vi "Find all UI Control Type Classes.vi"(4 "Label Black List":string[](array[string]), 5 "Reset to Defaults":bool, 6 "Label White List":string[](array[string]), 7 "Tab Label in Tag?":bool, 8 "error in (no error)":errorcluster, 9 "Root Label":string, 10 "Ctl Refnum":refnum<vi>, 11 "VI in":refnum<vi>) -> (0 "error out":errorcluster, 1 "Labels":string[](array[string]), 3 "Values":refnum<class "Abs_Type.lvclass">[](array[class]))   [LabVIEW 2021, in "UI-Bus.lvclass"]
uses:
  UI-Bus.lvclass
  <vilib>/TSA/Abstract Data Classes/Abs_Types/Type/Abs_Type.lvclass
  Support/Boolean/UI-Bus_Boolean.lvclass
  C:/Program Files (x86)/National Instruments/LabVIEW 2021/vi.lib/TSA/Abstract Data Classes/Abs_Types/Type/Abs_Type.lvclass
  C:/Program Files (x86)/National Instruments/LabVIEW 2021/vi.lib/TSA/Abstract Data Classes/Abs_Types/Value/Abs_Value.lvclass
  Support/U8/UI-Bus_U8.lvclass
  C:/Program Files (x86)/National Instruments/LabVIEW 2021/vi.lib/TSA/Abstract Data Classes/Abs_Types/Numeric/Abs_Numeric.lvclass
  Support/U16/UI-Bus_U16.lvclass
  Support/U32/UI-Bus_U32.lvclass
  Support/U64/UI-Bus_U64.lvclass
  Support/I8/UI-Bus_I8.lvclass
  Support/I16/UI-Bus_I16.lvclass
  Support/I32/UI-Bus_I32.lvclass
  Support/I64/UI-Bus_I64.lvclass
  Support/Single/UI-Bus_Single.lvclass
  Support/Double/UI-Bus_Double.lvclass
  Support/Extended/UI-Bus_Extended.lvclass
  Support/Complex Single/UI-Bus_ComplexSingle.lvclass
  Support/Complex Double/UI-Bus_ComplexDouble.lvclass
  Support/Complex Extended/UI-Bus_ComplexExtended.lvclass
  Support/Time/UI-Bus_Time.lvclass
  Support/String/UI-Bus_String.lvclass
  Support/Variant/UI-Bus_Variant.lvclass
  <vilib>/TSA/Abstract Data Classes/Abs_Types/Numeric/Abs_Numeric.lvclass
  <vilib>/Utility/Data Type/NI_Data Type.lvlib
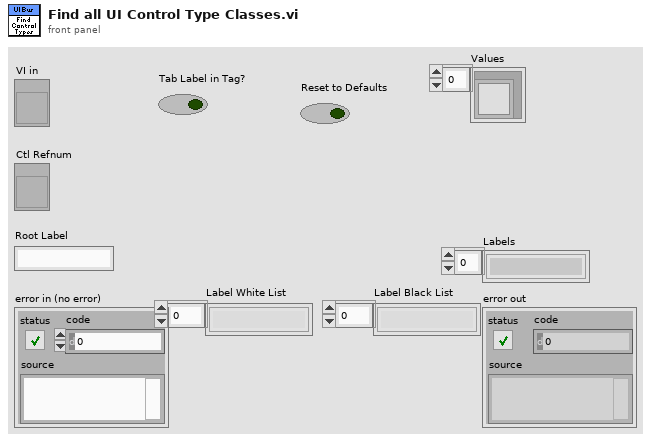
[diagram p1: front panel]
types:
  T1 = typedef "NI_Data Type.lvlib/Data Type.ctl" = enum8{"Invalid Type", "Void", "I8", "I16", "I32", "I64", "U8", "U16", "U32", "U64", "Single Float", "Double Float", "Extended Float", "Single Complex", "Double Complex", "Extended Complex", "Enum U8", "Enum U16", "Enum U32", "Enum U64", "Single Float With Unit", "Double Float With Unit", "Extended Float With Unit", "Single Complex with Unit", "Double Complex with Unit", "Extended Complex with Unit", "Boolean", "String", "Path", "Picture", "Tag", "Array", "Cluster", "Variant", "LV Variant", "Waveform", "Timestamp", "Digital Waveform", "Digital Data", "ExpressData", "Refnum", "External Data", "VI", "Poly VI", "LabVIEW Class Instance", "Fixed Point", "Set Collection", "Map Collection"}
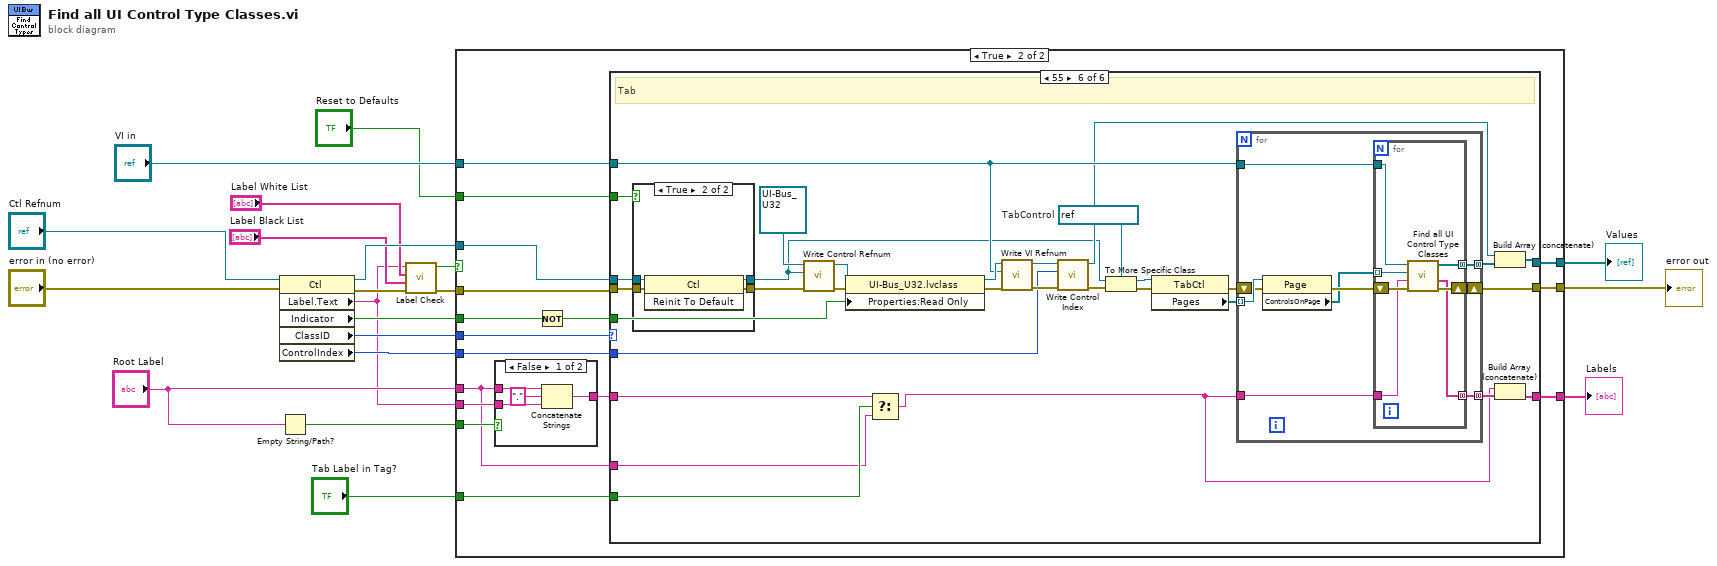
[diagram p0: block diagram]
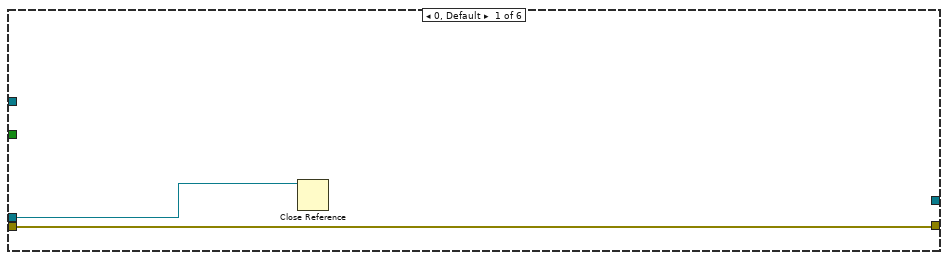
[diagram p4: hidden frame]
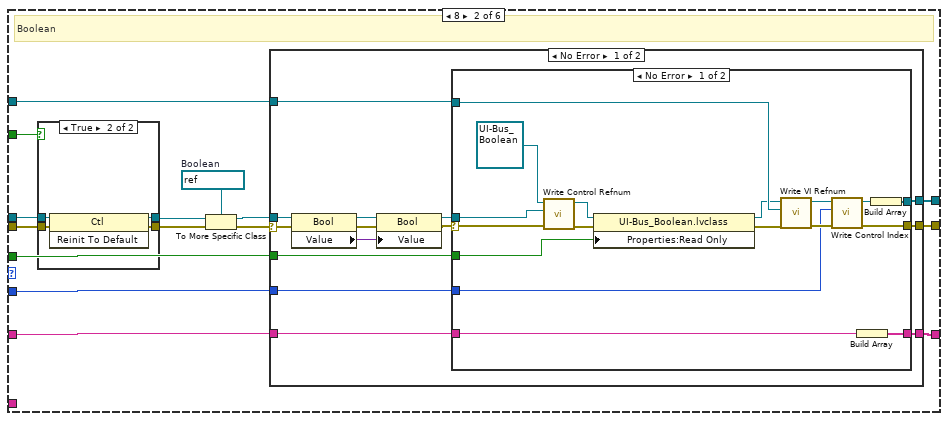
[diagram p5: hidden frame]
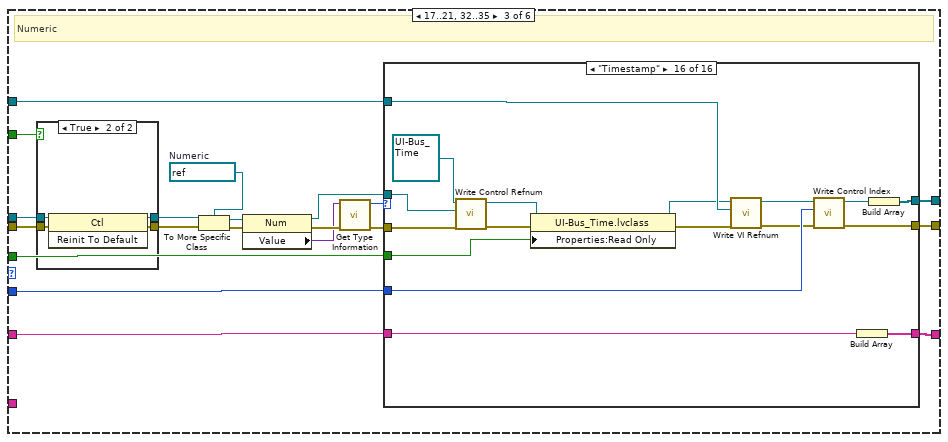
[diagram p9: hidden frame]
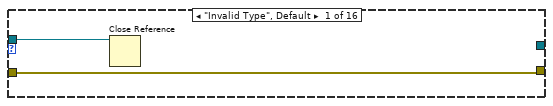
[diagram p11: hidden frame]
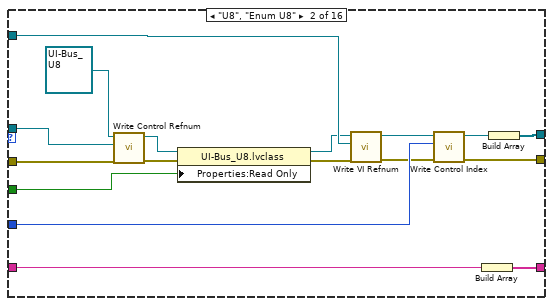
[diagram p12: hidden frame]
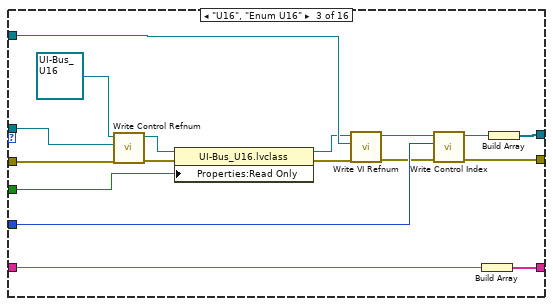
[diagram p13: hidden frame]
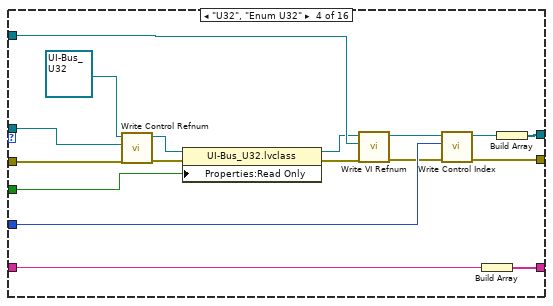
[diagram p14: hidden frame]
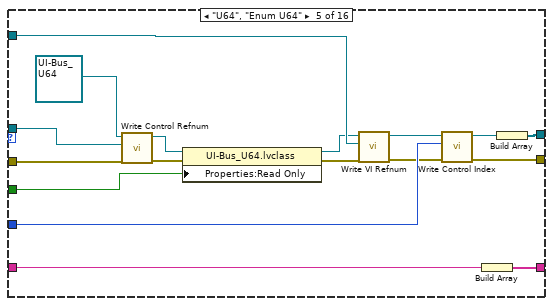
[diagram p15: hidden frame]
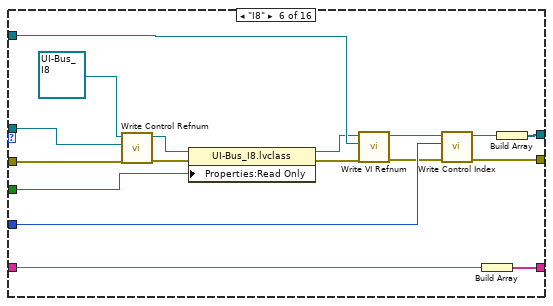
[diagram p16: hidden frame]
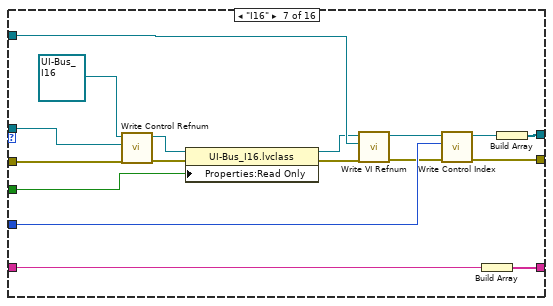
[diagram p17: hidden frame]
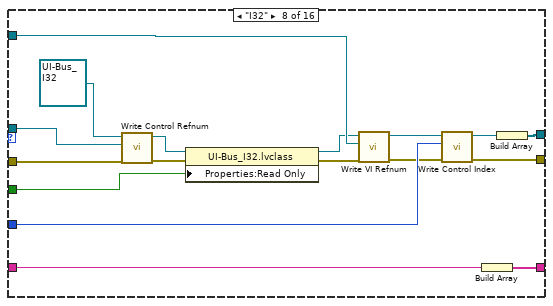
[diagram p18: hidden frame]
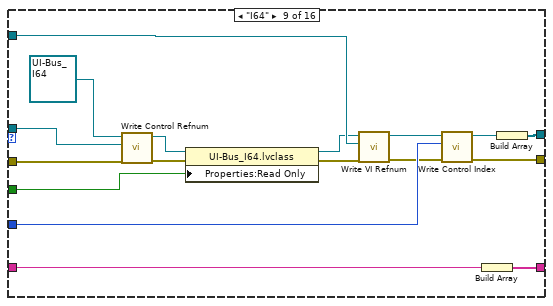
[diagram p19: hidden frame]
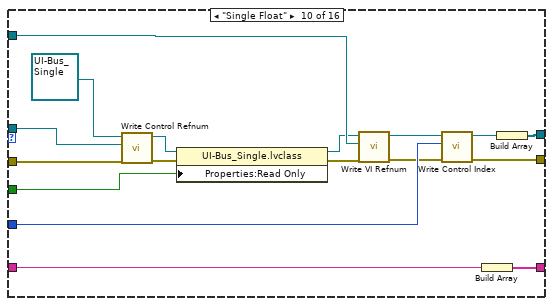
[diagram p20: hidden frame]
diagram:
  n1 = property class="Ctl"(reference="Ctl Refnum", error in="error in (no error)") -> (reference out=w19:refnum<vi>, error out=w11:errorcluster, "Label.Text"=w4:string, "Indicator"=w12:bool, "ClassID"=w13:u32, "ControlIndex"=w18:i32)
  n2 = Empty String/Path?(string/path="Root Label") -> (empty?=w15:bool)
  n3 = call "Label Check.vi"("error in (no error)"=w11, "Label Black List"="Label Black List", "Label White List"="Label White List", "Label"=w4) -> ("error out"=w10:errorcluster, "OK"=w9:bool)  [unwired: 6 in]
  n4 = case shown="True" w9 {
    tunnel: [w21 w37] -> w20
    tunnel: [_ w36] -> w5
    tunnel: w19 -> [_ w35]
    tunnel: w18 -> [_ w34]
    tunnel: "VI in" -> [_ w33]
    tunnel: [_ w32] -> w16
    tunnel: w15 -> [_ w31]
    tunnel: "Root Label" -> [_ w23]
    tunnel: w13 -> [_ w29]
    tunnel: w12 -> [_ w28]
    tunnel: w10 -> [w21 w26]
    tunnel: w4 -> [_ w24]
    tunnel: "Tab Label in Tag?" -> [_ w25]
    tunnel: "Reset to Defaults" -> [_ w22]
    frame False {
    }
    frame True {
      n5 = case shown="False" w31 {
        tunnel: w24 -> [w39 w42]
        tunnel: [w40 w42] -> w30
        tunnel: w23 -> [w38 _]
        frame False {
          n6 = Concatenate Strings(w38, "." ("string"), w39) -> (w40:string)
        }
        frame True {
        }
      }
      n7 = Not(x=w28) -> (.not. x?=w27:bool)
      n8 = case shown="55" w29 {
        tunnel: w26 -> [w44 w49 w102 w385 w411 w439]
        tunnel: w33 -> [_ w59 w117 w400 w426 w443]
        tunnel: w34 -> [_ w58 w116 w399 w425 w442]
        tunnel: w35 -> [w43 w48 w101 w384 w410 w438]
        tunnel: [_ w57 w115 w398 w424 w441] -> w36
        tunnel: [w44 w54 w112 w395 w421 w457] -> w37
        tunnel: w30 -> [_ w56 w114 w397 w423 w455]
        tunnel: [_ w55 w113 w396 w422 w434] -> w32
        tunnel: w27 -> [_ w53 w111 w394 w420 w444]
        tunnel: w25 -> [_ _ _ _ _ w454]
        tunnel: w23 -> [_ _ _ _ _ w453]
        tunnel: w22 -> [_ w45 w98 w381 w407 w435]
        frame 0, Default {
          n9 = Close Reference(reference=w43) -> ()  [unwired: 1 in, 1 out]
        }
        frame 8 {
          w52 = refnum<vi> refnum  # Boolean
          # "Boolean"
          n10 = case shown="True" w45 {
            tunnel: w49 -> [w60 w65]
            tunnel: w48 -> [w61 w64]
            tunnel: [w60 w63] -> w47
            tunnel: [w61 w62] -> w46
            frame False {
            }
            frame True {
              n11 = invoke class="Ctl" method="Reinit To Default"(reference=w64, error in=w65) -> (reference out=w62:refnum<vi>, error out=w63:errorcluster)  [unwired: 1 in, 1 out]
            }
          }
          n12 = To More Specific Class(target class=w52, reference=w46, error in=w47) -> (specific class reference=w50:refnum<vi>, error out=w51:errorcluster)
          n13 = case shown="No Error" w51 {
            selector: w51 -> [w70 w97]
            tunnel: w59 -> [w79 _]
            tunnel: w58 -> [w78 _]
            tunnel: [w77 _] -> w57
            tunnel: w56 -> [w76 _]
            tunnel: [w75 _] -> w55
            tunnel: [w74 w97] -> w54
            tunnel: w53 -> [w73 _]
            tunnel: w50 -> [w69 _]
            frame No Error {
              n14 = property class="Bool"(reference=w69, error in=w70) -> (reference out=w67:refnum<vi>, error out=w68:errorcluster, "Value"=w66:variant)
              n15 = property class="Bool"(reference=w67, error in=w68, "Value"=w66) -> (reference out=w72:refnum<vi>, error out=w71:errorcluster)
              n16 = case shown="No Error" w71 {
                selector: w71 -> [w80 _]
                tunnel: w79 -> [w96 _]
                tunnel: w78 -> [w93 _]
                tunnel: [w92 _] -> w77
                tunnel: w76 -> [w91 _]
                tunnel: [w90 _] -> w75
                tunnel: [w89 _] -> w74
                tunnel: w73 -> [w82 _]
                tunnel: w72 -> [w81 _]
                frame No Error {
                  n17 = call-dynamic "Write Control Refnum.vi"("error in (no error)"=w80, "Ctl Refnum"=w81, "UI-Bus_Boolean in"=refnum<class "UI-Bus_Boolean.lvclass"> refnum ("UI-Bus_Boolean.lvclass")) -> ("error out"=w86:errorcluster, "UI-Bus_Boolean out"=w84:refnum<class "UI-Bus_Boolean.lvclass">)  [unwired: 7 in]
                  n18 = property class="UI-Bus_Boolean.lvclass"(reference=w84, error in=w86, "Properties:Read Only"=w82) -> (reference out=w83:refnum<class "UI-Bus_Boolean.lvclass">, error out=w85:errorcluster)
                  n19 = call-dynamic "Write VI Refnum.vi"("error in (no error)"=w85, "VI Refnum"=w96, "UI-Bus_Boolean in"=w83) -> ("error out"=w95:errorcluster, "UI-Bus_Boolean out"=w94:refnum<class "UI-Bus_Boolean.lvclass">)  [unwired: 7 in]
                  n20 = call-dynamic "Write Control Index.vi"("error in (no error)"=w95, "Control Index"=w93, "UI-Bus_Boolean in"=w94) -> ("error out"=w89:errorcluster, "UI-Bus_Boolean out"=w88:refnum<class "UI-Bus_Boolean.lvclass">)  [unwired: 7 in]
                  n21 = Build Array(w91) -> (w90:string[])
                  n22 = Build Array(w88) -> (w92:refnum<class "UI-Bus_Boolean.lvclass">[])
                }
                frame Error {
                  # "If the boolean has a latching action then a reading from it will error"
                }
              }
            }
            frame Error {
            }
          }
        }
        frame 17..21, 32..35 {
          w110 = refnum<vi> refnum  # Numeric
          # "Numeric"
          n23 = case shown="True" w98 {
            tunnel: w102 -> [w118 w123]
            tunnel: w101 -> [w119 w122]
            tunnel: [w118 w121] -> w100
            tunnel: [w119 w120] -> w99
            frame False {
            }
            frame True {
              n24 = invoke class="Ctl" method="Reinit To Default"(reference=w122, error in=w123) -> (reference out=w120:refnum<vi>, error out=w121:errorcluster)  [unwired: 1 in, 1 out]
            }
          }
          n25 = To More Specific Class(target class=w110, reference=w99, error in=w100) -> (specific class reference=w108:refnum<vi>, error out=w109:errorcluster)
          n26 = property class="Num"(reference=w108, error in=w109) -> (reference out=w105:refnum<vi>, error out=w107:errorcluster, "Value"=w106:variant)
          n27 = call <vilib>:"Get Type Information.vi"("error in (no error)"=w107, "variant"=w106) -> ("error out"=w103:errorcluster, "type"=w104:T1)  [unwired: 5 in, 3 out]
          n28 = case shown="\"Timestamp\"" w104 {
            tunnel: w117 -> [_ w142 w159 w176 w193 w210 w227 w244 w261 w278 w295 w312 w329 w346 w363 w380]
            tunnel: w116 -> [_ w141 w158 w175 w192 w209 w226 w243 w260 w277 w294 w311 w328 w345 w362 w379]
            tunnel: [_ w140 w157 w174 w191 w208 w225 w242 w259 w276 w293 w310 w327 w344 w361 w378] -> w115
            tunnel: w114 -> [_ w139 w156 w173 w190 w207 w224 w241 w258 w275 w292 w309 w326 w343 w360 w377]
            tunnel: [_ w138 w155 w172 w189 w206 w223 w240 w257 w274 w291 w308 w325 w342 w359 w376] -> w113
            tunnel: [w125 w137 w154 w171 w188 w205 w222 w239 w256 w273 w290 w307 w324 w341 w358 w375] -> w112
            tunnel: w111 -> [_ w136 w153 w170 w187 w204 w221 w238 w255 w272 w289 w306 w323 w340 w357 w374]
            tunnel: w105 -> [w124 w127 w145 w162 w179 w196 w213 w230 w247 w264 w281 w298 w315 w332 w349 w366]
            tunnel: w103 -> [w125 w126 w144 w161 w178 w195 w212 w229 w246 w263 w280 w297 w314 w331 w348 w365]
            frame "Invalid Type", Default {
              n29 = Close Reference(reference=w124) -> ()  [unwired: 1 in, 1 out]
            }
            frame "U8", "Enum U8" {
              n30 = call-dynamic "Write Control Refnum.vi"("error in (no error)"=w126, "Ctl Refnum"=w127, "UI-Bus_Boolean in"=refnum<class "UI-Bus_U8.lvclass"> refnum ("UI-Bus_U8.lvclass")) -> ("error out"=w132:errorcluster, "UI-Bus_Boolean out"=w130:refnum<class "UI-Bus_U8.lvclass">)  [unwired: 7 in]
              n31 = property class="UI-Bus_U8.lvclass"(reference=w130, error in=w132, "Properties:Read Only"=w136) -> (reference out=w129:refnum<class "UI-Bus_U8.lvclass">, error out=w131:errorcluster)
              n32 = call-dynamic "Write VI Refnum.vi"("error in (no error)"=w131, "VI Refnum"=w142, "UI-Bus_Boolean in"=w129) -> ("error out"=w135:errorcluster, "UI-Bus_Boolean out"=w134:refnum<class "UI-Bus_U8.lvclass">)  [unwired: 7 in]
              n33 = call-dynamic "Write Control Index.vi"("error in (no error)"=w135, "Control Index"=w141, "UI-Bus_Boolean in"=w134) -> ("error out"=w137:errorcluster, "UI-Bus_Boolean out"=w133:refnum<class "UI-Bus_U8.lvclass">)  [unwired: 7 in]
              n34 = Build Array(w139) -> (w138:string[])
              n35 = Build Array(w133) -> (w140:refnum<class "UI-Bus_U8.lvclass">[])
            }
            frame "U16", "Enum U16" {
              n36 = call-dynamic "Write Control Refnum.vi"("error in (no error)"=w144, "Ctl Refnum"=w145, "UI-Bus_Boolean in"=refnum<class "UI-Bus_U16.lvclass"> refnum ("UI-Bus_U16.lvclass")) -> ("error out"=w149:errorcluster, "UI-Bus_Boolean out"=w147:refnum<class "UI-Bus_U16.lvclass">)  [unwired: 7 in]
              n37 = property class="UI-Bus_U16.lvclass"(reference=w147, error in=w149, "Properties:Read Only"=w153) -> (reference out=w146:refnum<class "UI-Bus_U16.lvclass">, error out=w148:errorcluster)
              n38 = call-dynamic "Write VI Refnum.vi"("error in (no error)"=w148, "VI Refnum"=w159, "UI-Bus_Boolean in"=w146) -> ("error out"=w152:errorcluster, "UI-Bus_Boolean out"=w151:refnum<class "UI-Bus_U16.lvclass">)  [unwired: 7 in]
              n39 = call-dynamic "Write Control Index.vi"("error in (no error)"=w152, "Control Index"=w158, "UI-Bus_Boolean in"=w151) -> ("error out"=w154:errorcluster, "UI-Bus_Boolean out"=w150:refnum<class "UI-Bus_U16.lvclass">)  [unwired: 7 in]
              n40 = Build Array(w156) -> (w155:string[])
              n41 = Build Array(w150) -> (w157:refnum<class "UI-Bus_U16.lvclass">[])
            }
            frame "U32", "Enum U32" {
              n42 = call-dynamic "Write Control Refnum.vi"("error in (no error)"=w161, "Ctl Refnum"=w162, "UI-Bus_Boolean in"=refnum<class "UI-Bus_U32.lvclass"> refnum ("UI-Bus_U32.lvclass")) -> ("error out"=w166:errorcluster, "UI-Bus_Boolean out"=w164:refnum<class "UI-Bus_U32.lvclass">)  [unwired: 7 in]
              n43 = property class="UI-Bus_U32.lvclass"(reference=w164, error in=w166, "Properties:Read Only"=w170) -> (reference out=w163:refnum<class "UI-Bus_U32.lvclass">, error out=w165:errorcluster)
              n44 = call-dynamic "Write VI Refnum.vi"("error in (no error)"=w165, "VI Refnum"=w176, "UI-Bus_Boolean in"=w163) -> ("error out"=w169:errorcluster, "UI-Bus_Boolean out"=w168:refnum<class "UI-Bus_U32.lvclass">)  [unwired: 7 in]
              n45 = call-dynamic "Write Control Index.vi"("error in (no error)"=w169, "Control Index"=w175, "UI-Bus_Boolean in"=w168) -> ("error out"=w171:errorcluster, "UI-Bus_Boolean out"=w167:refnum<class "UI-Bus_U32.lvclass">)  [unwired: 7 in]
              n46 = Build Array(w173) -> (w172:string[])
              n47 = Build Array(w167) -> (w174:refnum<class "UI-Bus_U32.lvclass">[])
            }
            frame "U64", "Enum U64" {
              n48 = call-dynamic "Write Control Refnum.vi"("error in (no error)"=w178, "Ctl Refnum"=w179, "UI-Bus_Boolean in"=refnum<class "UI-Bus_U64.lvclass"> refnum ("UI-Bus_U64.lvclass")) -> ("error out"=w183:errorcluster, "UI-Bus_Boolean out"=w181:refnum<class "UI-Bus_U64.lvclass">)  [unwired: 7 in]
              n49 = property class="UI-Bus_U64.lvclass"(reference=w181, error in=w183, "Properties:Read Only"=w187) -> (reference out=w180:refnum<class "UI-Bus_U64.lvclass">, error out=w182:errorcluster)
              n50 = call-dynamic "Write VI Refnum.vi"("error in (no error)"=w182, "VI Refnum"=w193, "UI-Bus_Boolean in"=w180) -> ("error out"=w186:errorcluster, "UI-Bus_Boolean out"=w185:refnum<class "UI-Bus_U64.lvclass">)  [unwired: 7 in]
              n51 = call-dynamic "Write Control Index.vi"("error in (no error)"=w186, "Control Index"=w192, "UI-Bus_Boolean in"=w185) -> ("error out"=w188:errorcluster, "UI-Bus_Boolean out"=w184:refnum<class "UI-Bus_U64.lvclass">)  [unwired: 7 in]
              n52 = Build Array(w190) -> (w189:string[])
              n53 = Build Array(w184) -> (w191:refnum<class "UI-Bus_U64.lvclass">[])
            }
            frame "I8" {
              n54 = call-dynamic "Write Control Refnum.vi"("error in (no error)"=w195, "Ctl Refnum"=w196, "UI-Bus_Boolean in"=refnum<class "UI-Bus_I8.lvclass"> refnum ("UI-Bus_I8.lvclass")) -> ("error out"=w200:errorcluster, "UI-Bus_Boolean out"=w198:refnum<class "UI-Bus_I8.lvclass">)  [unwired: 7 in]
              n55 = property class="UI-Bus_I8.lvclass"(reference=w198, error in=w200, "Properties:Read Only"=w204) -> (reference out=w197:refnum<class "UI-Bus_I8.lvclass">, error out=w199:errorcluster)
              n56 = call-dynamic "Write VI Refnum.vi"("error in (no error)"=w199, "VI Refnum"=w210, "UI-Bus_Boolean in"=w197) -> ("error out"=w203:errorcluster, "UI-Bus_Boolean out"=w202:refnum<class "UI-Bus_I8.lvclass">)  [unwired: 7 in]
              n57 = call-dynamic "Write Control Index.vi"("error in (no error)"=w203, "Control Index"=w209, "UI-Bus_Boolean in"=w202) -> ("error out"=w205:errorcluster, "UI-Bus_Boolean out"=w201:refnum<class "UI-Bus_I8.lvclass">)  [unwired: 7 in]
              n58 = Build Array(w207) -> (w206:string[])
              n59 = Build Array(w201) -> (w208:refnum<class "UI-Bus_I8.lvclass">[])
            }
            frame "I16" {
              n60 = call-dynamic "Write Control Refnum.vi"("error in (no error)"=w212, "Ctl Refnum"=w213, "UI-Bus_Boolean in"=refnum<class "UI-Bus_I16.lvclass"> refnum ("UI-Bus_I16.lvclass")) -> ("error out"=w217:errorcluster, "UI-Bus_Boolean out"=w215:refnum<class "UI-Bus_I16.lvclass">)  [unwired: 7 in]
              n61 = property class="UI-Bus_I16.lvclass"(reference=w215, error in=w217, "Properties:Read Only"=w221) -> (reference out=w214:refnum<class "UI-Bus_I16.lvclass">, error out=w216:errorcluster)
              n62 = call-dynamic "Write VI Refnum.vi"("error in (no error)"=w216, "VI Refnum"=w227, "UI-Bus_Boolean in"=w214) -> ("error out"=w220:errorcluster, "UI-Bus_Boolean out"=w219:refnum<class "UI-Bus_I16.lvclass">)  [unwired: 7 in]
              n63 = call-dynamic "Write Control Index.vi"("error in (no error)"=w220, "Control Index"=w226, "UI-Bus_Boolean in"=w219) -> ("error out"=w222:errorcluster, "UI-Bus_Boolean out"=w218:refnum<class "UI-Bus_I16.lvclass">)  [unwired: 7 in]
              n64 = Build Array(w224) -> (w223:string[])
              n65 = Build Array(w218) -> (w225:refnum<class "UI-Bus_I16.lvclass">[])
            }
            frame "I32" {
              n66 = call-dynamic "Write Control Refnum.vi"("error in (no error)"=w229, "Ctl Refnum"=w230, "UI-Bus_Boolean in"=refnum<class "UI-Bus_I32.lvclass"> refnum ("UI-Bus_I32.lvclass")) -> ("error out"=w234:errorcluster, "UI-Bus_Boolean out"=w232:refnum<class "UI-Bus_I32.lvclass">)  [unwired: 7 in]
              n67 = property class="UI-Bus_I32.lvclass"(reference=w232, error in=w234, "Properties:Read Only"=w238) -> (reference out=w231:refnum<class "UI-Bus_I32.lvclass">, error out=w233:errorcluster)
              n68 = call-dynamic "Write VI Refnum.vi"("error in (no error)"=w233, "VI Refnum"=w244, "UI-Bus_Boolean in"=w231) -> ("error out"=w237:errorcluster, "UI-Bus_Boolean out"=w236:refnum<class "UI-Bus_I32.lvclass">)  [unwired: 7 in]
              n69 = call-dynamic "Write Control Index.vi"("error in (no error)"=w237, "Control Index"=w243, "UI-Bus_Boolean in"=w236) -> ("error out"=w239:errorcluster, "UI-Bus_Boolean out"=w235:refnum<class "UI-Bus_I32.lvclass">)  [unwired: 7 in]
              n70 = Build Array(w241) -> (w240:string[])
              n71 = Build Array(w235) -> (w242:refnum<class "UI-Bus_I32.lvclass">[])
            }
            frame "I64" {
              n72 = call-dynamic "Write Control Refnum.vi"("error in (no error)"=w246, "Ctl Refnum"=w247, "UI-Bus_Boolean in"=refnum<class "UI-Bus_I64.lvclass"> refnum ("UI-Bus_I64.lvclass")) -> ("error out"=w251:errorcluster, "UI-Bus_Boolean out"=w249:refnum<class "UI-Bus_I64.lvclass">)  [unwired: 7 in]
              n73 = property class="UI-Bus_I64.lvclass"(reference=w249, error in=w251, "Properties:Read Only"=w255) -> (reference out=w248:refnum<class "UI-Bus_I64.lvclass">, error out=w250:errorcluster)
              n74 = call-dynamic "Write VI Refnum.vi"("error in (no error)"=w250, "VI Refnum"=w261, "UI-Bus_Boolean in"=w248) -> ("error out"=w254:errorcluster, "UI-Bus_Boolean out"=w253:refnum<class "UI-Bus_I64.lvclass">)  [unwired: 7 in]
              n75 = call-dynamic "Write Control Index.vi"("error in (no error)"=w254, "Control Index"=w260, "UI-Bus_Boolean in"=w253) -> ("error out"=w256:errorcluster, "UI-Bus_Boolean out"=w252:refnum<class "UI-Bus_I64.lvclass">)  [unwired: 7 in]
              n76 = Build Array(w258) -> (w257:string[])
              n77 = Build Array(w252) -> (w259:refnum<class "UI-Bus_I64.lvclass">[])
            }
            frame "Single Float" {
              n78 = call-dynamic "Write Control Refnum.vi"("error in (no error)"=w263, "Ctl Refnum"=w264, "UI-Bus_Boolean in"=refnum<class "UI-Bus_Single.lvclass"> refnum ("UI-Bus_Single.lvclass")) -> ("error out"=w268:errorcluster, "UI-Bus_Boolean out"=w266:refnum<class "UI-Bus_Single.lvclass">)  [unwired: 7 in]
              n79 = property class="UI-Bus_Single.lvclass"(reference=w266, error in=w268, "Properties:Read Only"=w272) -> (reference out=w265:refnum<class "UI-Bus_Single.lvclass">, error out=w267:errorcluster)
              n80 = call-dynamic "Write VI Refnum.vi"("error in (no error)"=w267, "VI Refnum"=w278, "UI-Bus_Boolean in"=w265) -> ("error out"=w271:errorcluster, "UI-Bus_Boolean out"=w270:refnum<class "UI-Bus_Single.lvclass">)  [unwired: 7 in]
              n81 = call-dynamic "Write Control Index.vi"("error in (no error)"=w271, "Control Index"=w277, "UI-Bus_Boolean in"=w270) -> ("error out"=w273:errorcluster, "UI-Bus_Boolean out"=w269:refnum<class "UI-Bus_Single.lvclass">)  [unwired: 7 in]
              n82 = Build Array(w275) -> (w274:string[])
              n83 = Build Array(w269) -> (w276:refnum<class "UI-Bus_Single.lvclass">[])
            }
            frame "Double Float" {
              n84 = call-dynamic "Write Control Refnum.vi"("error in (no error)"=w280, "Ctl Refnum"=w281, "UI-Bus_Boolean in"=refnum<class "UI-Bus_Double.lvclass"> refnum ("UI-Bus_Double.lvclass")) -> ("error out"=w285:errorcluster, "UI-Bus_Boolean out"=w283:refnum<class "UI-Bus_Double.lvclass">)  [unwired: 7 in]
              n85 = property class="UI-Bus_Double.lvclass"(reference=w283, error in=w285, "Properties:Read Only"=w289) -> (reference out=w282:refnum<class "UI-Bus_Double.lvclass">, error out=w284:errorcluster)
              n86 = call-dynamic "Write VI Refnum.vi"("error in (no error)"=w284, "VI Refnum"=w295, "UI-Bus_Boolean in"=w282) -> ("error out"=w288:errorcluster, "UI-Bus_Boolean out"=w287:refnum<class "UI-Bus_Double.lvclass">)  [unwired: 7 in]
              n87 = call-dynamic "Write Control Index.vi"("error in (no error)"=w288, "Control Index"=w294, "UI-Bus_Boolean in"=w287) -> ("error out"=w290:errorcluster, "UI-Bus_Boolean out"=w286:refnum<class "UI-Bus_Double.lvclass">)  [unwired: 7 in]
              n88 = Build Array(w292) -> (w291:string[])
              n89 = Build Array(w286) -> (w293:refnum<class "UI-Bus_Double.lvclass">[])
            }
            frame "Extended Float" {
              n90 = call-dynamic "Write Control Refnum.vi"("error in (no error)"=w297, "Ctl Refnum"=w298, "UI-Bus_Boolean in"=refnum<class "UI-Bus_Extended.lvclass"> refnum ("UI-Bus_Extended.lvclass")) -> ("error out"=w302:errorcluster, "UI-Bus_Boolean out"=w300:refnum<class "UI-Bus_Extended.lvclass">)  [unwired: 7 in]
              n91 = property class="UI-Bus_Extended.lvclass"(reference=w300, error in=w302, "Properties:Read Only"=w306) -> (reference out=w299:refnum<class "UI-Bus_Extended.lvclass">, error out=w301:errorcluster)
              n92 = call-dynamic "Write VI Refnum.vi"("error in (no error)"=w301, "VI Refnum"=w312, "UI-Bus_Boolean in"=w299) -> ("error out"=w305:errorcluster, "UI-Bus_Boolean out"=w304:refnum<class "UI-Bus_Extended.lvclass">)  [unwired: 7 in]
              n93 = call-dynamic "Write Control Index.vi"("error in (no error)"=w305, "Control Index"=w311, "UI-Bus_Boolean in"=w304) -> ("error out"=w307:errorcluster, "UI-Bus_Boolean out"=w303:refnum<class "UI-Bus_Extended.lvclass">)  [unwired: 7 in]
              n94 = Build Array(w309) -> (w308:string[])
              n95 = Build Array(w303) -> (w310:refnum<class "UI-Bus_Extended.lvclass">[])
            }
            frame "Single Complex" {
              n96 = call-dynamic "Write Control Refnum.vi"("error in (no error)"=w314, "Ctl Refnum"=w315, "UI-Bus_Boolean in"=refnum<class "UI-Bus_ComplexSingle.lvclass"> refnum ("UI-Bus_ComplexSingle.lvclass")) -> ("error out"=w319:errorcluster, "UI-Bus_Boolean out"=w317:refnum<class "UI-Bus_ComplexSingle.lvclass">)  [unwired: 7 in]
              n97 = property class="UI-Bus_ComplexSingle.lvclass"(reference=w317, error in=w319, "Properties:Read Only"=w323) -> (reference out=w316:refnum<class "UI-Bus_ComplexSingle.lvclass">, error out=w318:errorcluster)
              n98 = call-dynamic "Write VI Refnum.vi"("error in (no error)"=w318, "VI Refnum"=w329, "UI-Bus_Boolean in"=w316) -> ("error out"=w322:errorcluster, "UI-Bus_Boolean out"=w321:refnum<class "UI-Bus_ComplexSingle.lvclass">)  [unwired: 7 in]
              n99 = call-dynamic "Write Control Index.vi"("error in (no error)"=w322, "Control Index"=w328, "UI-Bus_Boolean in"=w321) -> ("error out"=w324:errorcluster, "UI-Bus_Boolean out"=w320:refnum<class "UI-Bus_ComplexSingle.lvclass">)  [unwired: 7 in]
              n100 = Build Array(w326) -> (w325:string[])
              n101 = Build Array(w320) -> (w327:refnum<class "UI-Bus_ComplexSingle.lvclass">[])
            }
            frame "Double Complex" {
              n102 = call-dynamic "Write Control Refnum.vi"("error in (no error)"=w331, "Ctl Refnum"=w332, "UI-Bus_Boolean in"=refnum<class "UI-Bus_ComplexDouble.lvclass"> refnum ("UI-Bus_ComplexDouble.lvclass")) -> ("error out"=w336:errorcluster, "UI-Bus_Boolean out"=w334:refnum<class "UI-Bus_ComplexDouble.lvclass">)  [unwired: 7 in]
              n103 = property class="UI-Bus_ComplexDouble.lvclass"(reference=w334, error in=w336, "Properties:Read Only"=w340) -> (reference out=w333:refnum<class "UI-Bus_ComplexDouble.lvclass">, error out=w335:errorcluster)
              n104 = call-dynamic "Write VI Refnum.vi"("error in (no error)"=w335, "VI Refnum"=w346, "UI-Bus_Boolean in"=w333) -> ("error out"=w339:errorcluster, "UI-Bus_Boolean out"=w338:refnum<class "UI-Bus_ComplexDouble.lvclass">)  [unwired: 7 in]
              n105 = call-dynamic "Write Control Index.vi"("error in (no error)"=w339, "Control Index"=w345, "UI-Bus_Boolean in"=w338) -> ("error out"=w341:errorcluster, "UI-Bus_Boolean out"=w337:refnum<class "UI-Bus_ComplexDouble.lvclass">)  [unwired: 7 in]
              n106 = Build Array(w343) -> (w342:string[])
              n107 = Build Array(w337) -> (w344:refnum<class "UI-Bus_ComplexDouble.lvclass">[])
            }
            frame "Extended Complex" {
              n108 = call-dynamic "Write Control Refnum.vi"("error in (no error)"=w348, "Ctl Refnum"=w349, "UI-Bus_Boolean in"=refnum<class "UI-Bus_ComplexExtended.lvclass"> refnum ("UI-Bus_ComplexExtended.lvclass")) -> ("error out"=w353:errorcluster, "UI-Bus_Boolean out"=w351:refnum<class "UI-Bus_ComplexExtended.lvclass">)  [unwired: 7 in]
              n109 = property class="UI-Bus_ComplexExtended.lvclass"(reference=w351, error in=w353, "Properties:Read Only"=w357) -> (reference out=w350:refnum<class "UI-Bus_ComplexExtended.lvclass">, error out=w352:errorcluster)
              n110 = call-dynamic "Write VI Refnum.vi"("error in (no error)"=w352, "VI Refnum"=w363, "UI-Bus_Boolean in"=w350) -> ("error out"=w356:errorcluster, "UI-Bus_Boolean out"=w355:refnum<class "UI-Bus_ComplexExtended.lvclass">)  [unwired: 7 in]
              n111 = call-dynamic "Write Control Index.vi"("error in (no error)"=w356, "Control Index"=w362, "UI-Bus_Boolean in"=w355) -> ("error out"=w358:errorcluster, "UI-Bus_Boolean out"=w354:refnum<class "UI-Bus_ComplexExtended.lvclass">)  [unwired: 7 in]
              n112 = Build Array(w360) -> (w359:string[])
              n113 = Build Array(w354) -> (w361:refnum<class "UI-Bus_ComplexExtended.lvclass">[])
            }
            frame "Timestamp" {
              n114 = call-dynamic "Write Control Refnum.vi"("error in (no error)"=w365, "Ctl Refnum"=w366, "UI-Bus_Boolean in"=refnum<class "UI-Bus_Time.lvclass"> refnum ("UI-Bus_Time.lvclass")) -> ("error out"=w370:errorcluster, "UI-Bus_Boolean out"=w368:refnum<class "UI-Bus_Time.lvclass">)  [unwired: 7 in]
              n115 = property class="UI-Bus_Time.lvclass"(reference=w368, error in=w370, "Properties:Read Only"=w374) -> (reference out=w367:refnum<class "UI-Bus_Time.lvclass">, error out=w369:errorcluster)
              n116 = call-dynamic "Write VI Refnum.vi"("error in (no error)"=w369, "VI Refnum"=w380, "UI-Bus_Boolean in"=w367) -> ("error out"=w373:errorcluster, "UI-Bus_Boolean out"=w372:refnum<class "UI-Bus_Time.lvclass">)  [unwired: 7 in]
              n117 = call-dynamic "Write Control Index.vi"("error in (no error)"=w373, "Control Index"=w379, "UI-Bus_Boolean in"=w372) -> ("error out"=w375:errorcluster, "UI-Bus_Boolean out"=w371:refnum<class "UI-Bus_Time.lvclass">)  [unwired: 7 in]
              n118 = Build Array(w377) -> (w376:string[])
              n119 = Build Array(w371) -> (w378:refnum<class "UI-Bus_Time.lvclass">[])
            }
          }
        }
        frame 27, 29 {
          # "String"
          n120 = case shown="True" w381 {
            tunnel: w385 -> [w401 w406]
            tunnel: w384 -> [w402 w405]
            tunnel: [w401 w404] -> w383
            tunnel: [w402 w403] -> w382
            frame False {
            }
            frame True {
              n121 = invoke class="Ctl" method="Reinit To Default"(reference=w405, error in=w406) -> (reference out=w403:refnum<vi>, error out=w404:errorcluster)  [unwired: 1 in, 1 out]
            }
          }
          n122 = call-dynamic "Write Control Refnum.vi"("error in (no error)"=w383, "Ctl Refnum"=w382, "UI-Bus_Boolean in"=refnum<class "UI-Bus_String.lvclass"> refnum ("UI-Bus_String.lvclass")) -> ("error out"=w390:errorcluster, "UI-Bus_Boolean out"=w388:refnum<class "UI-Bus_String.lvclass">)  [unwired: 7 in]
          n123 = property class="UI-Bus_String.lvclass"(reference=w388, error in=w390, "Properties:Read Only"=w394) -> (reference out=w387:refnum<class "UI-Bus_String.lvclass">, error out=w389:errorcluster)
          n124 = call-dynamic "Write VI Refnum.vi"("error in (no error)"=w389, "VI Refnum"=w400, "UI-Bus_Boolean in"=w387) -> ("error out"=w393:errorcluster, "UI-Bus_Boolean out"=w392:refnum<class "UI-Bus_String.lvclass">)  [unwired: 7 in]
          n125 = call-dynamic "Write Control Index.vi"("error in (no error)"=w393, "Control Index"=w399, "UI-Bus_Boolean in"=w392) -> ("error out"=w395:errorcluster, "UI-Bus_Boolean out"=w391:refnum<class "UI-Bus_String.lvclass">)  [unwired: 7 in]
          n126 = Build Array(w391) -> (w398:refnum<class "UI-Bus_String.lvclass">[])
          n127 = Build Array(w397) -> (w396:string[])
        }
        frame 10 {
          # "Variant"
          n128 = case shown="True" w407 {
            tunnel: w411 -> [w427 w432]
            tunnel: w410 -> [w428 w431]
            tunnel: [w427 w430] -> w409
            tunnel: [w428 w429] -> w408
            frame False {
            }
            frame True {
              n129 = invoke class="Ctl" method="Reinit To Default"(reference=w431, error in=w432) -> (reference out=w429:refnum<vi>, error out=w430:errorcluster)  [unwired: 1 in, 1 out]
            }
          }
          n130 = call-dynamic "Write Control Refnum.vi"("error in (no error)"=w409, "Ctl Refnum"=w408, "UI-Bus_Boolean in"=refnum<class "UI-Bus_Variant.lvclass"> refnum ("UI-Bus_Variant.lvclass")) -> ("error out"=w416:errorcluster, "UI-Bus_Boolean out"=w414:refnum<class "UI-Bus_Variant.lvclass">)  [unwired: 7 in]
          n131 = property class="UI-Bus_Variant.lvclass"(reference=w414, error in=w416, "Properties:Read Only"=w420) -> (reference out=w413:refnum<class "UI-Bus_Variant.lvclass">, error out=w415:errorcluster)
          n132 = call-dynamic "Write VI Refnum.vi"("error in (no error)"=w415, "VI Refnum"=w426, "UI-Bus_Boolean in"=w413) -> ("error out"=w419:errorcluster, "UI-Bus_Boolean out"=w418:refnum<class "UI-Bus_Variant.lvclass">)  [unwired: 7 in]
          n133 = call-dynamic "Write Control Index.vi"("error in (no error)"=w419, "Control Index"=w425, "UI-Bus_Boolean in"=w418) -> ("error out"=w421:errorcluster, "UI-Bus_Boolean out"=w417:refnum<class "UI-Bus_Variant.lvclass">)  [unwired: 7 in]
          n134 = Build Array(w417) -> (w424:refnum<class "UI-Bus_Variant.lvclass">[])
          n135 = Build Array(w423) -> (w422:string[])
        }
        frame 55 {
          w463 = refnum<vi> refnum  # TabControl
          # "Tab"
          n136 = case shown="True" w435 {
            tunnel: w439 -> [w464 w469]
            tunnel: w438 -> [w465 w468]
            tunnel: [w464 w467] -> w436
            tunnel: [w465 w466] -> w437
            frame False {
            }
            frame True {
              n137 = invoke class="Ctl" method="Reinit To Default"(reference=w468, error in=w469) -> (reference out=w466:refnum<vi>, error out=w467:errorcluster)  [unwired: 1 in, 1 out]
            }
          }
          n138 = call-dynamic "Write Control Refnum.vi"("error in (no error)"=w436, "Ctl Refnum"=w437, "UI-Bus_Boolean in"=refnum<class "UI-Bus_U32.lvclass"> refnum ("UI-Bus_U32.lvclass")) -> ("error out"=w449:errorcluster, "UI-Bus_Boolean out"=w451:refnum<class "UI-Bus_U32.lvclass">)  [unwired: 7 in]
          n139 = property class="UI-Bus_U32.lvclass"(reference=w451, error in=w449, "Properties:Read Only"=w444) -> (reference out=w452:refnum<class "UI-Bus_U32.lvclass">, error out=w450:errorcluster)
          n140 = Select(t=w455, s=w454, f=w453) -> (s? t:f=w433:string)
          n141 = call-dynamic "Write VI Refnum.vi"("error in (no error)"=w450, "VI Refnum"=w443, "UI-Bus_Boolean in"=w452) -> ("error out"=w447:errorcluster, "UI-Bus_Boolean out"=w448:refnum<class "UI-Bus_U32.lvclass">)  [unwired: 7 in]
          n142 = call-dynamic "Write Control Index.vi"("error in (no error)"=w447, "Control Index"=w442, "UI-Bus_Boolean in"=w448) -> ("error out"=w445:errorcluster, "UI-Bus_Boolean out"=w440:refnum<class "UI-Bus_U32.lvclass">)  [unwired: 7 in]
          n143 = To More Specific Class(target class=w463, reference=w437, error in=w445) -> (specific class reference=w462:refnum<vi>, error out=w461:errorcluster)
          n144 = property class="TabCtl"(reference=w462, error in=w461) -> (error out=w459:errorcluster, "Pages"=w460:refnum<vi>[])  [unwired: 1 out]
          n145 = for {
            tunnel: w460 -> [w478] mode=indexing
            shift-right: [w470] -> w457
            shift-left: w459 -> [w477]
            tunnel: w433 -> [w476]
            tunnel: [w473] -> w456 mode=concatenating
            tunnel: w443 -> [w472]
            tunnel: [w471] -> w458 mode=concatenating
            n146 = property class="Page"(reference=w478, error in=w477) -> (error out=w475:errorcluster, "ControlsOnPage"=w474:refnum<vi>[])  [unwired: 1 out]
            n147 = for {
              tunnel: w474 -> [w484] mode=indexing
              tunnel: w476 -> [w480]
              tunnel: [w479] -> w473 mode=concatenating
              shift-right: [w482] -> w470
              shift-left: w475 -> [w485]
              tunnel: w472 -> [w483]
              tunnel: [w481] -> w471 mode=concatenating
              n148 = call "Find all UI Control Type Classes.vi"("error in (no error)"=w485, "Root Label"=w480, "Ctl Refnum"=w484, "VI in"=w483) -> ("error out"=w482:errorcluster, "Labels"=w479:string[], "Values"=w481:refnum<class "Abs_Type.lvclass">[])  [unwired: 5 in]
            }
          }
          n149 = Build Array (concatenate)(w440, w458) -> (w441:refnum<class "Abs_Type.lvclass">[])
          n150 = Build Array (concatenate)(w433, w456) -> (w434:string[])
        }
      }
    }
  }
  "error out" <- w20
  "Labels" <- w16
  "Values" <- w5
